vi "RH_SCOPE_Initialize.vi"(8 "error in":errorcluster, 11 "SCOPE Resource Name":refnum<k15>) -> (0 "error out":errorcluster, 3 "SCOPE Session Out":refnum<k15>)   [LabVIEW 2023, in "ResourceHandling.lvlib"]
doc: "Initialize Scope resource"
uses:
  ResourceHandling.lvlib
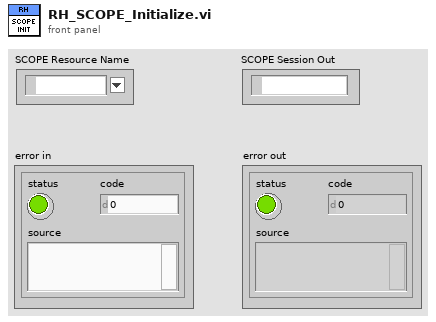
[diagram p1: front panel]
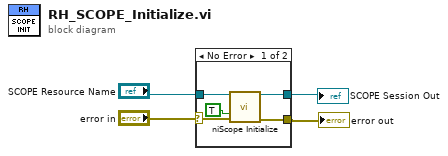
[diagram p0: block diagram]
diagram:
  n1 = case shown="No Error" "error in" {
    selector: "error in" -> [w6 w10]
    tunnel: [w7 w10] -> w3
    tunnel: [w9 w11] -> w4
    tunnel: "SCOPE Resource Name" -> [w8 w11]
    frame No Error {
      n2 = call <instrlib>:"niScope Initialize.vi"("resource name"=w8, "reset device"=TRUE, "error in"=w6) -> ("instrument handle"=w9:refnum<k15>, "error out"=w7:errorcluster)  [unwired: 11 in]
    }
    frame Error {
    }
  }
  "error out" <- w3
  "SCOPE Session Out" <- w4
